vi "update.vi"(8 "error in (no error)":errorcluster, 11 "TrajectoryAK101022Resonance in":refnum<class "TrajectoryAK101022Resonance.lvclass">) -> (0 "error out":errorcluster, 3 "TrajectoryAK101022Resonance out":refnum<class "TrajectoryAK101022Resonance.lvclass">)   [LabVIEW 2010, in "TrajectoryAK101022Resonance.lvclass"]
uses:
  TrajectoryAK101022Resonance.lvclass
  FPGAWrapper/FPGAWrapperAK101022Resonance/FPGAWrapperAK101022Resonance/FPGAWrapperAK101022Resonance.lvclass
  FPGAWrapper/GenericFPGAWrapper/GenericFPGAWrapper/GenericFPGAWrapper.lvclass
  FPGAWrapper/FPGAWrapperAK101022Resonance/scan_specification_cluster.ctl
  TrajectoryAK101022Resonance.lvclass/TrajectoryAK101022Resonance.ctl
  common/classes/GenericComponent/GenericComponent/class_data.vi
  common/classes/GenericComponent/GenericComponent/GenericComponent.lvclass
panel:
  out "Waveform Graph":u32[](graph)
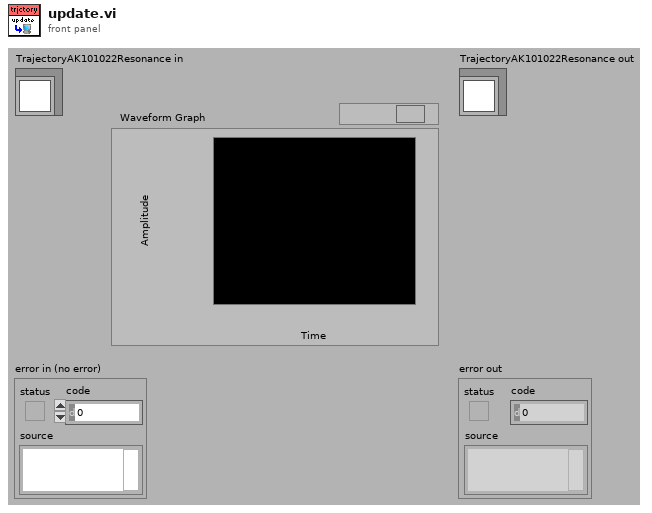
[diagram p1: front panel]
types:
  T1 = typedef "scan_specification_cluster.ctl" = cluster{"x amplitude":u16, "x resolution (pixels)":u16, "x offset fly-forward (iterations)":u16, "x offset fly-back (iterations)":u16, "y resolution (nr. of lines)":u16, "y step size":u16, "iterations per pixel":u16, "number of frames":i32, "y offset (pixels)":u16, "number of y-brake lines  (before y-fly-back)":u16, "number y-brake lines (after y-fly-back)":u16, "number of y-fly-back steps":u16, "lines per z step":u16, "number of z/intensity tuples":u16, "number of repetitions (volumes or planes)":i32, "z step size derived":u16, "choose the beginning of z scan":bool, "number of frames (settings)":i32, "FPGA trajectory?":bool, "Pockels cell voltage (bits)":i16, "Vy min(bits)":i16, "Vz min(bits)":i16}
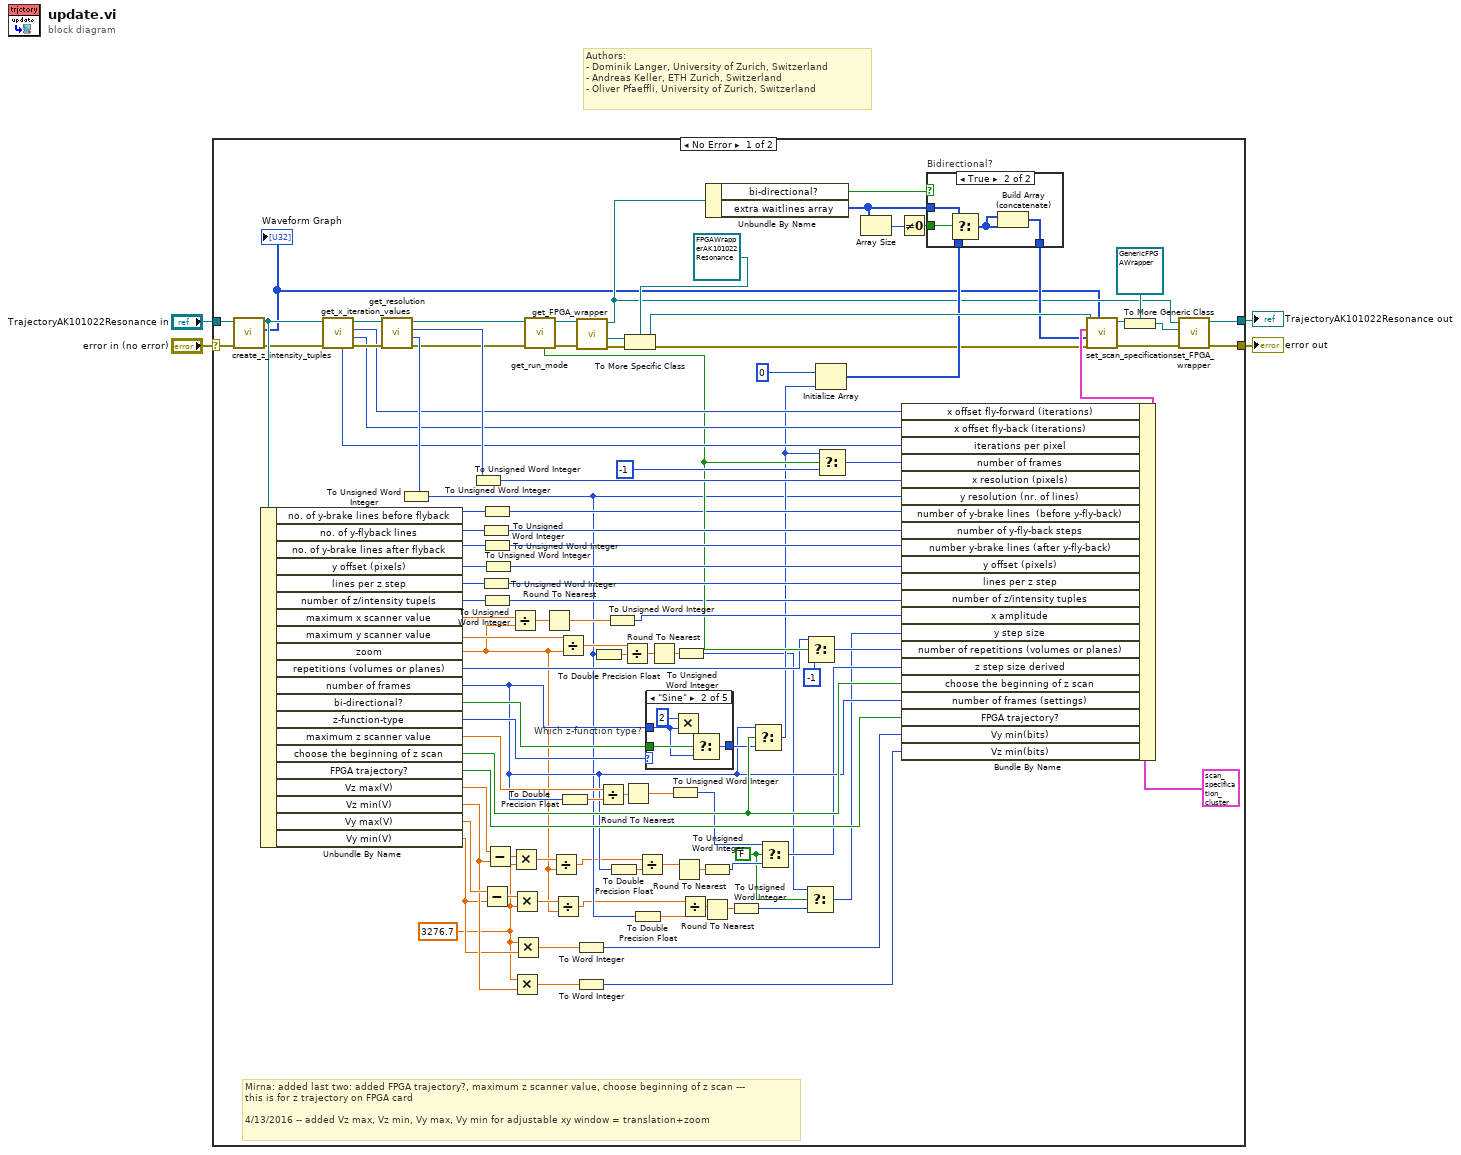
[diagram p0: block diagram]
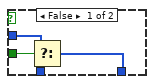
[diagram p2: hidden frame]
diagram:
  # "Authors: \n- Dominik Langer, University of Zurich, Switzerland\n- Andreas Keller, ETH Zurich, Switzerland\n- Oliver Pfaeffli, University of Zurich, Switzerland"
  n1 = case shown="No Error" "error in (no error)" {
    selector: "error in (no error)" -> [w58 w130]
    tunnel: "TrajectoryAK101022Resonance in" -> [w57 w129]
    tunnel: [w74 w130] -> w2
    tunnel: [w73 w129] -> w1
    frame No Error {
      w26 = FALSE ("s")
      w11 = 3276.7 ("y")
      # "Mirna: added last two: added FPGA trajectory?, maximum z scanner value, choose beginning of z scan ---\nthis is for z trajectory on FPGA card\n\n4/13/2016 -- added Vz max, Vz min, Vy max, Vy min for adjustable xy window = translation+zoom"
      n2 = call "create_z_intensity_tuples.vi"("error in (no error)"=w58, "TrajectoryAK101022Resonance in"=w57) -> ("error out"=w63:errorcluster, "z/intensity tuples"=w60:u32[], "TrajectoryAK101022Resonance out"=w64:refnum<class "TrajectoryAK101022Resonance.lvclass">)  [unwired: 7 in]
      "Waveform Graph" <- w60
      n3 = Unbundle By Name(w64) -> ("no. of y-brake lines before flyback"=w107:i32, "no. of y-flyback lines"=w106:i32, "no. of y-brake lines after flyback"=w105:i32, "y offset (pixels)"=w101:u16, "lines per z step"=w99:i32, "number of z/intensity tupels"=w97:i32, "maximum x scanner value"=w94:dbl, "maximum y scanner value"=w90:dbl, "zoom"=w5:dbl, "repetitions (volumes or planes)"=w48:i32, "number of frames"=w33:i32, "bi-directional?"=w71:bool, "z-function-type"=w37:enum16{"Sine", "tooth", "Stack", "Step"}, "maximum z scanner value"=w46:dbl, "choose the beginning of z scan"=w40:bool, "FPGA trajectory?"=w41:bool, "Vz max(V)"=w13:dbl, "Vz min(V)"=w17:dbl, "Vy max(V)"=w36:dbl, "Vy min(V)"=w12:dbl)
      n4 = call-dynamic "get_x_iteration_values.vi"("error in (no error)"=w63, "TrajectoryAK101022Resonance in"=w64) -> ("error out"=w87:errorcluster, "fly-back offset [iterations]"=w85:u16, "fly-forward offset [iterations]"=w86:u16, "TrajectoryAK101022Resonance out"=w88:refnum<class "TrajectoryAK101022Resonance.lvclass">, "iterations per pixel"=w84:u16)  [unwired: 4 in, 1 out]
      n5 = call-dynamic "get_resolution.vi"("error in (no error)"=w87, "TrajectoryAK101022Resonance in"=w88) -> ("error out"=w56:errorcluster, "y resolution"=w110:i32, "x resolution"=w109:i32, "TrajectoryAK101022Resonance out"=w55:refnum<class "TrajectoryAK101022Resonance.lvclass">)  [unwired: 6 in]
      n6 = To Unsigned Word Integer(number=w110) -> (unsigned 16bit integer=w23:u16)
      n7 = To Unsigned Word Integer(number=w109) -> (unsigned 16bit integer=w108:u16)
      n8 = To Unsigned Word Integer(number=w106) -> (unsigned 16bit integer=w103:u16)
      n9 = To Unsigned Word Integer(number=w99) -> (unsigned 16bit integer=w98:u16)
      n10 = To Unsigned Word Integer(number=w107) -> (unsigned 16bit integer=w42:u16)
      n11 = To Unsigned Word Integer(number=w105) -> (unsigned 16bit integer=w104:u16)
      n12 = To Unsigned Word Integer(number=w97) -> (unsigned 16bit integer=w47:u16)
      n13 = Subtract(x=w36, y=w12) -> (x-y=w35:dbl)
      n14 = To Unsigned Word Integer(number=w101) -> (unsigned 16bit integer=w100:u16)
      n15 = Subtract(x=w13, y=w17) -> (x-y=w34:dbl)
      n16 = Divide(x=w94, y=w5) -> (x/y=w95:dbl)
      n17 = Multiply(x=w34, y=w11) -> (x*y=w10:dbl)
      n18 = Multiply(x=w35, y=w11) -> (x*y=w7:dbl)
      n19 = Multiply(x=w11, y=w17) -> (x*y=w16:dbl)
      n20 = Multiply(x=w11, y=w12) -> (x*y=w18:dbl)
      n21 = call "get_run_mode.vi"("error in (no error)"=w56, "GenericPlugin in"=w55) -> ("error out"=w53:errorcluster, "GenericPlugin out"=w54:refnum<class "TrajectoryAK101022Resonance.lvclass">, "is NOT free run?"=w49:bool)  [unwired: 5 in, 2 out]
      n22 = Round To Nearest(number=w95) -> (nearest integer value=w96:dbl)
      n23 = Divide(x=w10, y=w5) -> (x/y=w9:dbl)
      n24 = Divide(x=w7, y=w5) -> (x/y=w6:dbl)
      n25 = Divide(x=w90, y=w5) -> (x/y=w93:dbl)
      n26 = To Double Precision Float(number=w33) -> (double precision float=w45:dbl)
      n27 = To Word Integer(number=w18) -> (16bit integer=w15:i16)
      n28 = To Word Integer(number=w16) -> (16bit integer=w14:i16)
      n29 = call-dynamic "get_FPGA_wrapper.vi"("error in (no error)"=w53, "TrajectoryMG100122GenericFPGA in"=w54) -> ("error out"=w75:errorcluster, "GenericFPGAWrapper.lvclass"=w81:refnum<class "GenericFPGAWrapper.lvclass">, "TrajectoryMG100122GenericFPGA out"=w61:refnum<class "TrajectoryAK101022Resonance.lvclass">)  [unwired: 7 in]
      n30 = To Double Precision Float(number=w23) -> (double precision float=w25:dbl)
      n31 = Divide(x=w46, y=w45) -> (x/y=w44:dbl)
      n32 = To Unsigned Word Integer(number=w96) -> (unsigned 16bit integer=w89:u16)
      n33 = To Double Precision Float(number=w33) -> (double precision float=w32:dbl)
      n34 = Divide(x=w93, y=w25) -> (x/y=w91:dbl)
      n35 = Round To Nearest(number=w44) -> (nearest integer value=w43:dbl)
      n36 = To More Specific Class(target class=refnum<class "FPGAWrapperAK101022Resonance.lvclass"> refnum ("FPGAWrapperAK101022Resonance.lvclass"), reference=w81, error in=w75) -> (specific class reference=w80:refnum<class "FPGAWrapperAK101022Resonance.lvclass">, error out=w62:errorcluster)
      n37 = To Double Precision Float(number=w23) -> (double precision float=w24:dbl)
      n38 = Divide(x=w9, y=w32) -> (x/y=w29:dbl)
      n39 = case "Which z-function type?" shown="\"Sine\"" w37 {
        tunnel: w71 -> [_ w125 _ _ _]
        tunnel: w33 -> [w120 w122 w126 w127 w128]
        tunnel: [w120 w121 w126 w127 w128] -> w39
        frame Default {
        }
        frame "Sine" {
          n40 = Multiply(x=2, y=w122) -> (x*y=w124:i32)
          n41 = Select(t=w124, s=w125, f=w122) -> (s? t:f=w121:i32)
        }
        frame "tooth" {
        }
        frame "Stack" {
        }
        frame "Step" {
        }
      }
      n42 = Round To Nearest(number=w91) -> (nearest integer value=w92:dbl)
      n43 = To Unsigned Word Integer(number=w43) -> (unsigned 16bit integer=w28:u16)
      n44 = Round To Nearest(number=w29) -> (nearest integer value=w31:dbl)
      n45 = To Unsigned Word Integer(number=w92) -> (unsigned 16bit integer=w8:u16)
      n46 = Divide(x=w6, y=w24) -> (x/y=w22:dbl)
      n47 = To Unsigned Word Integer(number=w31) -> (unsigned 16bit integer=w30:u16)
      n48 = Round To Nearest(number=w22) -> (nearest integer value=w21:dbl)
      n49 = Unbundle By Name(w61) -> ("bi-directional?"=w70:bool, "extra waitlines array"=w83:u32[])
      n50 = To Unsigned Word Integer(number=w21) -> (unsigned 16bit integer=w20:u16)
      n51 = Select(t=w33, s=w40, f=w39) -> (s? t:f=w38:i32)
      n52 = Select(t=w28, s=w26, f=w30) -> (s? t:f=w27:u16)
      n53 = Select(t=w8, s=w26, f=w20) -> (s? t:f=w19:u16)
      n54 = Select(t=w48, s=w49, f=-1 ("t")) -> (s? t:f=w59:i32)
      n55 = Initialize Array(u32 0 ("element"), w38) -> (w66:u32[])
      n56 = Select(t=w38, s=w49, f=-1 ("t")) -> (s? t:f=w50:i32)
      n57 = Array Size(array=w83) -> (size(s)=w69:i32)
      n58 = Not Equal To 0?(x=w69) -> (x != 0?=w67:bool)
      n59 = Bundle By Name(cluster=T1 {"x amplitude"=0, "x resolution (pixels)"=0, "x offset fly-forward (iterations)"=0, "x offset fly-back (iterations)"=0, "y resolution (nr. of lines)"=0, "y step size"=0, "iterations per pixel"=0, "number of frames"=0, "y offset (pixels)"=0, "number of y-brake lines  (before y-fly-back)"=0, "number y-brake lines (after y-fly-back)"=0, "number of y-fly-back steps"=0, "lines per z step"=0, "number of z/intensity tuples"=0, "number of repetitions (volumes or planes)"=0, "z step size derived"=0, "choose the beginning of z scan"=FALSE, "number of frames (settings)"=0, "FPGA trajectory?"=FALSE, "Pockels cell voltage (bits)"=0, "Vy min(bits)"=0, "Vz min(bits)"=0} ("scan specification"), "x offset fly-forward (iterations)"=w86, "x offset fly-back (iterations)"=w85, "iterations per pixel"=w84, "number of frames"=w50, "x resolution (pixels)"=w108, "y resolution (nr. of lines)"=w23, "number of y-brake lines  (before y-fly-back)"=w42, "number of y-fly-back steps"=w103, "number y-brake lines (after y-fly-back)"=w104, "y offset (pixels)"=w100, "lines per z step"=w98, "number of z/intensity tuples"=w47, "x amplitude"=w89, "y step size"=w19, "number of repetitions (volumes or planes)"=w59, "z step size derived"=w27, "choose the beginning of z scan"=w40, "number of frames (settings)"=w33, "FPGA trajectory?"=w41, "Vy min(bits)"=w15, "Vz min(bits)"=w14) -> (w72:T1)
      n60 = case "Bidirectional?" shown="True" w70 {
        tunnel: w67 -> [w114 w119]
        tunnel: w66 -> [w112 w118]
        tunnel: w83 -> [w113 w117]
        tunnel: [w111 w115] -> w65
        frame False {
          n61 = Select(t=w113, s=w114, f=w112) -> (s? t:f=w111:u32[])
        }
        frame True {
          n62 = Select(t=w117, s=w119, f=w118) -> (s? t:f=w116:u32[])
          n63 = Build Array (concatenate)(w116, w116) -> (w115:u32[])
        }
      }
      n64 = call-dynamic "set_scan_specification.vi"("z/intensity tuples (U32: high U16 is z, low U16 is intensity)"=w60, "error in (no error)"=w62, "extra waitlines array"=w65, "scan specification"=w72, "FPGA_AK101022Resonance in"=w80) -> ("error out"=w76:errorcluster, "FPGA_AK101022Resonance out"=w78:refnum<class "FPGAWrapperAK101022Resonance.lvclass">)  [unwired: 5 in]
      n65 = To More Generic Class(target class=refnum<class "GenericFPGAWrapper.lvclass"> refnum ("GenericFPGAWrapper.lvclass"), reference=w78) -> (generic class reference=w79:refnum<class "GenericFPGAWrapper.lvclass">)
      n66 = call-dynamic "set_FPGA_wrapper.vi"("error in (no error)"=w76, "GenericFPGAWrapper.lvclass"=w79, "TrajectoryMG100122GenericFPGA in"=w61) -> ("error out"=w74:errorcluster, "TrajectoryMG100122GenericFPGA out"=w73:refnum<class "TrajectoryAK101022Resonance.lvclass">)  [unwired: 7 in]
    }
    frame Error {
    }
  }
  "error out" <- w2
  "TrajectoryAK101022Resonance out" <- w1
